vi "Teleop.vi"(10 "Match Info":T1={"Autonomous Elapsed Seconds"=0.0, "TeleOp Elapsed Seconds"=0.0, "Disabled Elapsed Seconds"=0.0, "Visited Autonomous"=FALSE, "Visited TeleOp"=FALSE, "Visited Disabled"=FALSE, "Autonomous Settings"={"Autonomous Style"=enum."Independent", "VI Refnum"=refnum}}, 11 "Call Context":T2) -> ()   [LabVIEW 2013]
doc: "This VI is called for each TeleOp packet received from the DS where the robot is not disabled. It is often used to read from the joysticks and update I/O or to update setpoints for timed control loops. It should complete and return within 20 milliseconds or it may miss DS packets."
uses:
  <vilib>/Rock Robotics/WPI/DriverStation/WPI_DriverStationDerivedRobotMode.ctl
  <vilib>/Rock Robotics/WPI/DriverStation/WPI_DriverStationMatch Info.ctl
  Robot Global Data.vi
  <vilib>/Rock Robotics/WPI/Joystick/WPI_JoystickGetSetRefNum.vi
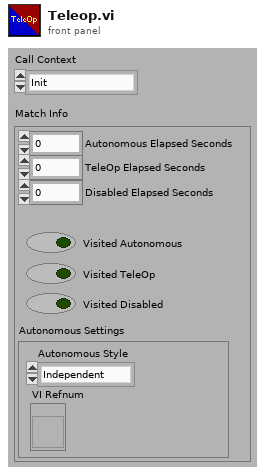
[diagram p1: front panel]
types:
  T1 = typedef "WPI_DriverStationMatch Info.ctl" = cluster{"Autonomous Elapsed Seconds":dbl, "TeleOp Elapsed Seconds":dbl, "Disabled Elapsed Seconds":dbl, "Visited Autonomous":bool, "Visited TeleOp":bool, "Visited Disabled":bool, "Autonomous Settings":cluster{"Autonomous Style":enum16{"Iterative", "Independent"}, "VI Refnum":refnum<vi>}}
  T2 = typedef "WPI_DriverStationDerivedRobotMode.ctl" = enum16{"Init", "Execute", "Stop"}
  T3 = typedef "WPI_JoystickDevRef.ctl" = cluster{"Device":T4}
  T4 = typedef "WPI_JoystickDeviceEnum.ctl" = enum16{"USB 1", "USB 2", "USB 3", "USB 4", "Kinect 1", "Kinect 2"}
  T5 = typedef "WPI_JoystickButtonState.ctl" = cluster{"Button 1":bool, "Button 2":bool, "Button 3":bool, "Button 4":bool, "Button 5":bool, "Button 6":bool, "Button 7":bool, "Button 8":bool, "Button 9":bool, "Button 10":bool, "Button 11":bool, "Button 12":bool}
  T6 = cluster{"axis 1 (x)":dbl, "axis 2 (y)":dbl, "axis 3 (throttle)":dbl, "axis 4":dbl, "axis 5":dbl, "axis 6":dbl}
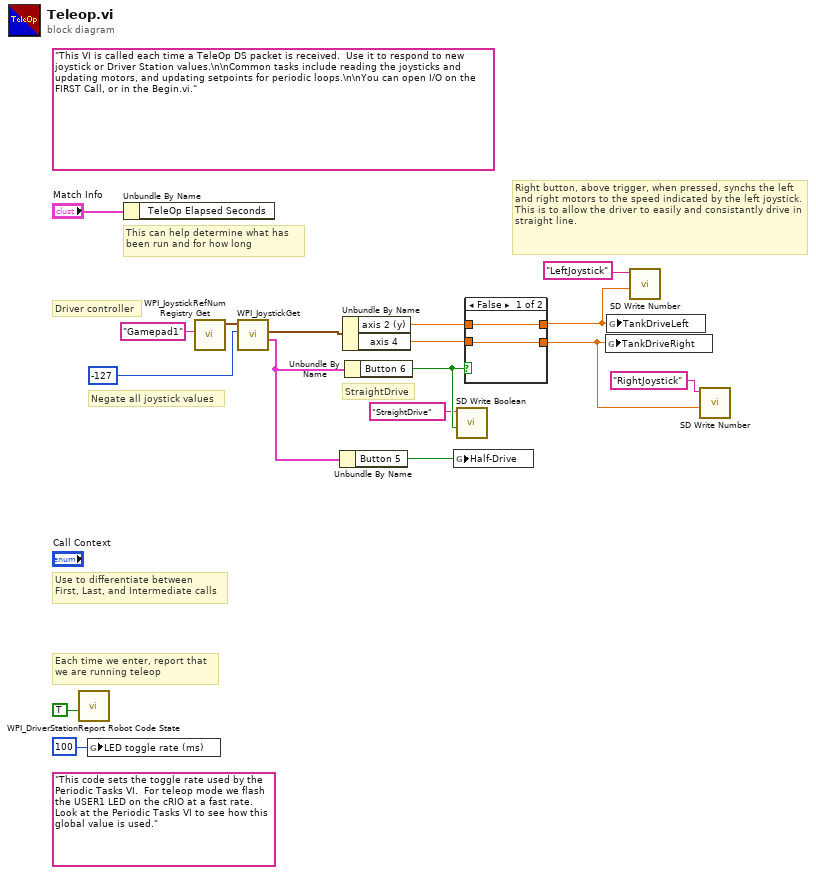
[diagram p0: block diagram]
diagram:
  (unwired) "This code sets the toggle rate used by the Periodic Tasks VI.  For teleop mode we flash the USER1 LED on the cRIO at a fast rate.  Look at the Periodic Tasks VI to see how this global value is used."
  (unwired) "This VI is called each time a TeleOp DS packet is received.  Use it to respond to new joystick or Driver Station values.\n\nCommon tasks include reading the joysticks and updating motors, and updating setpoints for periodic loops.\n\nYou can open I/O on the FIRST Call, or in the Begin.vi."
  # "StraightDrive"
  # "Right button, above trigger, when pressed, synchs the left and right motors to the speed indicated by the left joystick. This is to allow the driver to easily and consistantly drive in straight line."
  # "Negate all joystick values"
  # "Driver controller"
  # "Each time we enter, report that\nwe are running teleop"
  # "Use to differentiate between\nFirst, Last, and Intermediate calls"
  # "This can help determine what has\nbeen run and for how long"
  n1 = call <vilib>:"WPI_DriverStationReport Robot Code State.vi"("TeleOp"=TRUE ("Autonomous")) -> ()  [unwired: 10 in, 1 out]
  n2 = global write "Robot Global Data.vi" "LED toggle rate (ms)"(u32 100 ("LED ms toggle rate")) -> ()
  n3 = Unbundle By Name("Match Info") -> ()  [unwired: 1 out]
  n4 = call <vilib>:"WPI_JoystickRefNum Registry Get.vi"("refnum name"="Gamepad1") -> ("JoystickDevRef"=w14:T3)  [unwired: 1 in, 9 out]
  n5 = call <vilib>:"WPI_JoystickGet.vi"("Scaler"=i8 -127, "JoystickDevRef"=w14) -> ("Buttons"=w8:T5, "Axes"=w13:T6)  [unwired: 3 in, 1 out]
  n6 = Unbundle By Name(w8) -> ("Button 5"=w7:bool)
  n7 = Unbundle By Name(w13) -> ("axis 2 (y)"=w10:dbl, "axis 4"=w9:dbl)
  n8 = Unbundle By Name(w8) -> ("Button 6"=w6:bool)
  n9 = global write "Robot Global Data.vi" "Half-Drive"(w7) -> ()
  n10 = call <vilib>:"SD Write Boolean.vi"("Boolean"=w6, "Name"="StraightDrive") -> ()  [unwired: 8 in, 2 out]
  n11 = case shown="False" w6 {
    tunnel: w10 -> [w19 w20]
    tunnel: [w19 w20] -> w4
    tunnel: [w18 w20] -> w3
    tunnel: w9 -> [w18 _]
    frame False {
    }
    frame True {
    }
  }
  n12 = global write "Robot Global Data.vi" "TankDriveRight"(w3) -> ()
  n13 = global write "Robot Global Data.vi" "TankDriveLeft"(w4) -> ()
  n14 = call <vilib>:"SD Write Number.vi"("Numeric"=w4, "Name"="LeftJoystick") -> ()  [unwired: 8 in, 2 out]
  n15 = call <vilib>:"SD Write Number.vi"("Numeric"=w3, "Name"="RightJoystick") -> ()  [unwired: 8 in, 2 out]
